vi "STS_show.vi"() -> ()   [LabVIEW 2014]
uses:
  <userlib>/Nanonis Prog Interface V5/Nanonis Prog Interface.lvlib
  <vilib>/Analysis/NI_AALPro.lvlib
panel:
  in  "sub":bool
  in  "Filter order (2) 3":i32=2 min=1 max=1000 step=1
  in  "Filter type (none) 3":T1(ring)
  in  "Display (Y) off":u16(ring) items=["Y", "dY/dX", "dY/dX/(Y/X)"]
  in  "Datafile (1=last) 2":i32
  out "path out 2":path=path "D:/STM Data/092016/160908_16-21-42_STS001.dat"
  in  "Datafile (1=last)":i32
  out "x/y":dbl=-0.00010071572331476725 format="%#_6p"
  in  "fit":dbl=0.0040000000000000036 step=0.001 format="%#_6p"
  out "path out":path=path "D:/STM Data/092016/160908_16-21-42_STS001.dat"
  in  "Filter type pre":T1(ring)=enum."Gaussian"
  in  "Filter order pre":i32=1 min=1 max=1000 step=1
  in  "Ring":u16(ring)=1 items=["Bias calc (V)", "Current (A)", "LI Demod 1 X (A)", "LI Demod 1 Y (A)", "LI Demod 2 X (A)", "LI Demod 2 Y (A)", "Current [bwd] (A)", "LI Demod 1 X [bwd] (A)", "LI Demod 1 Y [bwd] (A)", "LI Demod 2 X [bwd] (A)", "LI Demod 2 Y [bwd] (A)", "Current (A) [filt]", "LI Demod 1 X (A) [filt]", "LI Demod 1 Y (A) [filt]", "LI Demod 2 X (A) [filt]", "LI Demod 2 Y (A) [filt]", "Current (A) [bwd] [filt]", "LI Demod 1 X (A) [bwd] [filt]", "LI Demod 1 Y (A) [bwd] [filt]", "LI Demod 2 X (A) [bwd] [filt]", "LI Demod 2 Y (A) [bwd] [filt]"]
  in  "Filter order (2) 2":i32=2 min=1 max=1000 step=1
  in  "Filter type (none) 2":T1(ring)
  in  "Cutoff frq (0.125) 2":dbl=0.125
  in  "Display (Y) 2":u16(ring)=1 items=["Y", "dY/dX", "dY/dX/(Y/X)"]
  in  "Filter type (none)":T1(ring)
  in  "Filter order (2)":i32=2 min=1 max=1000 step=1
  in  "Cutoff frq (0.125)":dbl=0.125
  in  "Display (Y)":u16(ring)=1 items=["Y", "dY/dX", "dY/dX/(Y/X)"]
  out "XY Graph 3":cluster{"X":dbl, "Y":dbl}[](graph)=[{"X"=-0.029999999329447746, "Y"=nan}, {"X"=-0.02939390018582344, "Y"=nan}, {"X"=-0.028787899762392044, "Y"=1.5525849362798114e-07}, {"X"=-0.02818180061876774, "Y"=5.168520876965395e-07}, {"X"=-0.027575800195336342, "Y"=-1.8705937225910675e-07}, {"X"=-0.026969699189066887, "Y"=-6.639889207903243e-07}, {"X"=-0.02636360004544258, "Y"=-9.874879833106362e-07}, {"X"=-0.025757599622011185, "Y"=-9.458443087316431e-07}, {"X"=-0.02515150047838688, "Y"=6.648643762964484e-07}, {"X"=-0.024545500054955482, "Y"=-4.47928062817252e-08}, {"X"=-0.023939400911331177, "Y"=-1.997370443932008e-06}, {"X"=-0.023333299905061722, "Y"=-2.2367739676225265e-06}, {"X"=-0.022727299481630325, "Y"=5.692607935118802e-07}, {"X"=-0.02212120033800602, "Y"=-1.5689885119641845e-06}, {"X"=-0.021515099331736565, "Y"=-2.758229187147329e-06}, {"X"=-0.020909100770950317, "Y"=-3.194582565724868e-06}, {"X"=-0.020302999764680862, "Y"=-5.236577534894633e-06}, {"X"=-0.019696999341249466, "Y"=-4.579991401925592e-06}, {"X"=-0.01909090019762516, "Y"=-1.7059288454535867e-06}, {"X"=-0.018484799191355705, "Y"=-5.031002994112464e-06}, {"X"=-0.017878800630569458, "Y"=-4.138250071188697e-06}, {"X"=-0.017272699624300003, "Y"=1.3100562902328957e-06}, {"X"=-0.016666699200868607, "Y"=5.068503950570972e-06}, {"X"=-0.0160606000572443, "Y"=4.011176770052973e-06}, {"X"=-0.01545449998229742, "Y"=2.537647009919699e-06}, {"X"=-0.014848499558866024, "Y"=5.116801095124242e-06}, {"X"=-0.014242400415241718, "Y"=1.6464771934735616e-07}, {"X"=-0.013636399991810322, "Y"=-3.0547176995608757e-06}, {"X"=-0.013030299916863441, "Y"=-5.217728993780238e-06}, {"X"=-0.012424199841916561, "Y"=-4.200614920252031e-06}, {"X"=-0.01181820034980774, "Y"=-6.242418446009756e-06}, {"X"=-0.011212100274860859, "Y"=-5.663095474505132e-06}, {"X"=-0.010606099851429462, "Y"=2.384088352720359e-06}, {"X"=-0.009999999776482582, "Y"=5.200079061493491e-06}, {"X"=-0.00939393974840641, "Y"=2.6398627367813077e-06}, {"X"=-0.008787879720330238, "Y"=6.452597551494918e-06}, {"X"=-0.008181819692254066, "Y"=1.2737566183337942e-05}, {"X"=-0.007575760129839182, "Y"=1.218992844152106e-05}, {"X"=-0.00696970010176301, "Y"=1.3279965824539184e-05}, {"X"=-0.006363640073686838, "Y"=1.1414322380559252e-05}, {"X"=-0.005757580045610666, "Y"=9.543383623890207e-06}, {"X"=-0.005151509772986174, "Y"=5.78405585714029e-06}, {"X"=-0.004545450210571289, "Y"=3.834239501672442e-06}, {"X"=-0.003939390182495117, "Y"=3.134550055729865e-06}, {"X"=-0.0033333299215883017, "Y"=1.0710322804966455e-06}, {"X"=-0.00272726989351213, "Y"=-8.661794169541851e-07}, {"X"=-0.0021212100982666016, "Y"=-1.4950962022879021e-06}, {"X"=-0.0015151499537751079, "Y"=-1.4481620816107035e-06}, {"X"=-0.0009090899839065969, "Y"=1.666731229290195e-07}, {"X"=-0.00030303001403808594, "Y"=-1.0913610732735875e-07}, {"X"=0.000303031993098557, "Y"=-1.1114294931287702e-06}, {"X"=0.0009090920211747289, "Y"=-1.284203208185384e-06}, {"X"=0.0015151499537751079, "Y"=6.035322429293407e-07}, {"X"=0.0021212100982666016, "Y"=4.756593350934117e-07}, {"X"=0.00272726989351213, "Y"=2.604464071554455e-07}, {"X"=0.0033333399333059788, "Y"=-1.6241975350996586e-09}, {"X"=0.003939399961382151, "Y"=-6.075334228327941e-07}, {"X"=0.0045454599894583225, "Y"=5.413411018824718e-07}, {"X"=0.005151520017534494, "Y"=-6.982397520424381e-07}, {"X"=0.005757580045610666, "Y"=-2.891121857582741e-06}, {"X"=0.006363640073686838, "Y"=-6.245094796472283e-06}, {"X"=0.00696970010176301, "Y"=-7.859388367794901e-06}, {"X"=0.007575760129839182, "Y"=-9.478467599884328e-06}, {"X"=0.008181819692254066, "Y"=-1.1359428289945348e-05}, {"X"=0.008787879720330238, "Y"=-1.258334103807099e-05}, {"X"=0.00939393974840641, "Y"=-9.133998297466377e-06}, {"X"=0.009999999776482582, "Y"=-8.996086304044726e-06}, {"X"=0.010606099851429462, "Y"=-7.816056623611081e-06}, {"X"=0.011212100274860859, "Y"=-2.158336854899807e-06}, {"X"=0.01181820034980774, "Y"=4.32424257909858e-06}, {"X"=0.012424199841916561, "Y"=2.8658121975906245e-06}, {"X"=0.013030299916863441, "Y"=2.6437646358981405e-06}, {"X"=0.013636399991810322, "Y"=5.652839123077133e-06}, {"X"=0.014242400415241718, "Y"=4.531496689082075e-06}, {"X"=0.014848499558866024, "Y"=3.876928205429419e-06}, {"X"=0.01545449998229742, "Y"=-8.604612293367695e-07}, {"X"=0.0160606000572443, "Y"=-4.179218333770935e-06}, {"X"=0.016666699200868607, "Y"=-4.138505304353997e-06}, {"X"=0.017272699624300003, "Y"=-7.2625928712624055e-06}, {"X"=0.017878800630569458, "Y"=-4.703849285510032e-06}, {"X"=0.018484799191355705, "Y"=-1.8761172247980886e-06}, {"X"=0.01909090019762516, "Y"=2.9486464571849516e-06}, {"X"=0.019696999341249466, "Y"=5.764776470791144e-06}, {"X"=0.020302999764680862, "Y"=3.1401164125217956e-06}, {"X"=0.020909100770950317, "Y"=5.540729187932117e-06}, {"X"=0.021515199914574623, "Y"=5.104789941335857e-06}, {"X"=0.02212120033800602, "Y"=3.022872010196525e-06}, {"X"=0.022727299481630325, "Y"=1.5019503969055098e-06}, {"X"=0.023333299905061722, "Y"=2.6840593826798465e-06}, {"X"=0.023939400911331177, "Y"=3.009385765408917e-06}, {"X"=0.024545500054955482, "Y"=6.751681966771312e-07}, {"X"=0.02515150047838688, "Y"=2.3592434760700652e-07}, {"X"=0.025757599622011185, "Y"=1.0180363796469083e-06}, {"X"=0.02636360004544258, "Y"=7.318487219108044e-07}, {"X"=0.026969699189066887, "Y"=7.621898569330085e-07}, {"X"=0.027575800195336342, "Y"=5.613791177103256e-07}, {"X"=0.02818180061876774, "Y"=-3.547310154327501e-07}, {"X"=0.028787899762392044, "Y"=4.214083566107483e-07}, {"X"=0.02939390018582344, "Y"=7.204319939562927e-07}, {"X"=0.029999999329447746, "Y"=8.404090983124726e-07}]
  out "XY Graph 2":cluster{"X":dbl, "Y":dbl}[](graph)=[{"X"=-0.029999999329447746, "Y"=nan}, {"X"=-0.02939390018582344, "Y"=3.391442095720389e-08}, {"X"=-0.028787899762392044, "Y"=3.400850767008377e-08}, {"X"=-0.02818180061876774, "Y"=3.432177127781708e-08}, {"X"=-0.027575800195336342, "Y"=3.420841321902125e-08}, {"X"=-0.026969699189066887, "Y"=3.380596886597846e-08}, {"X"=-0.02636360004544258, "Y"=3.320745324495459e-08}, {"X"=-0.025757599622011185, "Y"=3.263427119336304e-08}, {"X"=-0.02515150047838688, "Y"=3.3037244922462626e-08}, {"X"=-0.024545500054955482, "Y"=3.301010046288922e-08}, {"X"=-0.023939400911331177, "Y"=3.179949594732153e-08}, {"X"=-0.023333299905061722, "Y"=3.0443784994748196e-08}, {"X"=-0.022727299481630325, "Y"=3.078875727665929e-08}, {"X"=-0.02212120033800602, "Y"=2.983779468320142e-08}, {"X"=-0.021515099331736565, "Y"=2.8166029197349645e-08}, {"X"=-0.020909100770950317, "Y"=2.623011676020754e-08}, {"X"=-0.020302999764680862, "Y"=2.305622184689988e-08}, {"X"=-0.019696999341249466, "Y"=2.0280745118020816e-08}, {"X"=-0.01909090019762516, "Y"=1.9246783105707396e-08}, {"X"=-0.018484799191355705, "Y"=1.619748712843119e-08}, {"X"=-0.017878800630569458, "Y"=1.3689713541117256e-08}, {"X"=-0.017272699624300003, "Y"=1.4483739976897043e-08}, {"X"=-0.016666699200868607, "Y"=1.7555255517106758e-08}, {"X"=-0.0160606000572443, "Y"=1.9986426322361574e-08}, {"X"=-0.01545449998229742, "Y"=2.152449436526263e-08}, {"X"=-0.014848499558866024, "Y"=2.4625277995522153e-08}, {"X"=-0.014242400415241718, "Y"=2.472507083721828e-08}, {"X"=-0.013636399991810322, "Y"=2.287391061782101e-08}, {"X"=-0.013030299916863441, "Y"=1.9711444683638296e-08}, {"X"=-0.012424199841916561, "Y"=1.7165451665650556e-08}, {"X"=-0.01181820034980774, "Y"=1.3382549257837903e-08}, {"X"=-0.011212100274860859, "Y"=9.950146666309003e-09}, {"X"=-0.010606099851429462, "Y"=1.1394905217555401e-08}, {"X"=-0.009999999776482582, "Y"=1.454667352645631e-08}, {"X"=-0.00939393974840641, "Y"=1.614658881082723e-08}, {"X"=-0.008787879720330238, "Y"=2.0057250264050477e-08}, {"X"=-0.008181819692254066, "Y"=2.7776979982746367e-08}, {"X"=-0.007575760129839182, "Y"=3.516480267988338e-08}, {"X"=-0.00696970010176301, "Y"=4.32132591403542e-08}, {"X"=-0.006363640073686838, "Y"=5.0131023682786414e-08}, {"X"=-0.005757580045610666, "Y"=5.591488702982299e-08}, {"X"=-0.005151509772986174, "Y"=5.94204313400353e-08}, {"X"=-0.004545450210571289, "Y"=6.174420885461277e-08}, {"X"=-0.003939390182495117, "Y"=6.364393434939458e-08}, {"X"=-0.0033333299215883017, "Y"=6.4293044452752e-08}, {"X"=-0.00272726989351213, "Y"=6.376808773099374e-08}, {"X"=-0.0021212100982666016, "Y"=6.286197003276277e-08}, {"X"=-0.0015151499537751079, "Y"=6.198429671233468e-08}, {"X"=-0.0009090899839065969, "Y"=6.208531062019493e-08}, {"X"=-0.00030303001403808594, "Y"=6.201916759427655e-08}, {"X"=0.000303031993098557, "Y"=6.134557240488006e-08}, {"X"=0.0009090920211747289, "Y"=6.056726817247172e-08}, {"X"=0.0015151499537751079, "Y"=6.093304367587914e-08}, {"X"=0.0021212100982666016, "Y"=6.122132184123459e-08}, {"X"=0.00272726989351213, "Y"=6.137916793742765e-08}, {"X"=0.0033333399333059788, "Y"=6.137818355996292e-08}, {"X"=0.003939399961382151, "Y"=6.100998183666366e-08}, {"X"=0.0045454599894583225, "Y"=6.133806704006934e-08}, {"X"=0.005151520017534494, "Y"=6.09148918363426e-08}, {"X"=0.005757580045610666, "Y"=5.916269844216437e-08}, {"X"=0.006363640073686838, "Y"=5.537779611447602e-08}, {"X"=0.00696970010176301, "Y"=5.0614534979628706e-08}, {"X"=0.007575760129839182, "Y"=4.4870014639923725e-08}, {"X"=0.008181819692254066, "Y"=3.798552450123619e-08}, {"X"=0.008787879720330238, "Y"=3.035926447841084e-08}, {"X"=0.00939393974840641, "Y"=2.482351321380066e-08}, {"X"=0.009999999776482582, "Y"=1.9371344895795647e-08}, {"X"=0.010606099851429462, "Y"=1.463403239043591e-08}, {"X"=0.011212100274860859, "Y"=1.3326079342459039e-08}, {"X"=0.01181820034980774, "Y"=1.594700309373918e-08}, {"X"=0.012424199841916561, "Y"=1.7683683829958364e-08}, {"X"=0.013030299916863441, "Y"=1.928606977391814e-08}, {"X"=0.013636399991810322, "Y"=2.2712255990077847e-08}, {"X"=0.014242400415241718, "Y"=2.5458344902439555e-08}, {"X"=0.014848499558866024, "Y"=2.7808147767643243e-08}, {"X"=0.01545449998229742, "Y"=2.728670789831886e-08}, {"X"=0.0160606000572443, "Y"=2.475368335300092e-08}, {"X"=0.016666699200868607, "Y"=2.2245338832147316e-08}, {"X"=0.017272699624300003, "Y"=1.7844204476952457e-08}, {"X"=0.017878800630569458, "Y"=1.499319669166497e-08}, {"X"=0.018484799191355705, "Y"=1.385627235357104e-08}, {"X"=0.01909090019762516, "Y"=1.5643449938403702e-08}, {"X"=0.019696999341249466, "Y"=1.9137476020535762e-08}, {"X"=0.020302999764680862, "Y"=2.1040387896147848e-08}, {"X"=0.020909100770950317, "Y"=2.4398629432420044e-08}, {"X"=0.021515199914574623, "Y"=2.7492638244245676e-08}, {"X"=0.02212120033800602, "Y"=2.9324499962403687e-08}, {"X"=0.022727299481630325, "Y"=3.02348308117343e-08}, {"X"=0.023333299905061722, "Y"=3.18613719341533e-08}, {"X"=0.023939400911331177, "Y"=3.368536367482062e-08}, {"X"=0.024545500054955482, "Y"=3.4094582540629e-08}, {"X"=0.02515150047838688, "Y"=3.423755279517662e-08}, {"X"=0.025757599622011185, "Y"=3.4854583773059e-08}, {"X"=0.02636360004544258, "Y"=3.529808440842467e-08}, {"X"=0.026969699189066887, "Y"=3.57600470279909e-08}, {"X"=0.027575800195336342, "Y"=3.610029947613379e-08}, {"X"=0.02818180061876774, "Y"=3.588533233057729e-08}, {"X"=0.028787899762392044, "Y"=3.614074757463519e-08}, {"X"=0.02939390018582344, "Y"=3.657732966802623e-08}, {"X"=0.029999999329447746, "Y"=3.7086700902807496e-08}]
  out "XY Graph":cluster{"X":dbl, "Y":dbl}[](graph)=[{"X"=-0.029999999329447746, "Y"=-1.0017100482428987e-09}, {"X"=-0.02939390018582344, "Y"=-9.811545467442232e-10}, {"X"=-0.028787899762392044, "Y"=-9.605453766958825e-10}, {"X"=-0.02818180061876774, "Y"=-9.397429805167283e-10}, {"X"=-0.027575800195336342, "Y"=-9.190126676210852e-10}, {"X"=-0.026969699189066887, "Y"=-8.985228358735018e-10}, {"X"=-0.02636360004544258, "Y"=-8.783958268997907e-10}, {"X"=-0.025757599622011185, "Y"=-8.586194447382376e-10}, {"X"=-0.02515150047838688, "Y"=-8.385955988830266e-10}, {"X"=-0.024545500054955482, "Y"=-8.185914640250028e-10}, {"X"=-0.023939400911331177, "Y"=-7.993178167636466e-10}, {"X"=-0.023333299905061722, "Y"=-7.808658080436788e-10}, {"X"=-0.022727299481630325, "Y"=-7.622078080970968e-10}, {"X"=-0.02212120033800602, "Y"=-7.441231462919706e-10}, {"X"=-0.021515099331736565, "Y"=-7.270516876528421e-10}, {"X"=-0.020909100770950317, "Y"=-7.111562746469011e-10}, {"X"=-0.020302999764680862, "Y"=-6.971818753847233e-10}, {"X"=-0.019696999341249466, "Y"=-6.848917352556985e-10}, {"X"=-0.01909090019762516, "Y"=-6.732262764978065e-10}, {"X"=-0.018484799191355705, "Y"=-6.634089632502278e-10}, {"X"=-0.017878800630569458, "Y"=-6.551130165467347e-10}, {"X"=-0.017272699624300003, "Y"=-6.463344071721923e-10}, {"X"=-0.016666699200868607, "Y"=-6.356959148953792e-10}, {"X"=-0.0160606000572443, "Y"=-6.235821590172856e-10}, {"X"=-0.01545449998229742, "Y"=-6.105361613693062e-10}, {"X"=-0.014848499558866024, "Y"=-5.956132324769039e-10}, {"X"=-0.014242400415241718, "Y"=-5.806273882164156e-10}, {"X"=-0.013636399991810322, "Y"=-5.667657886964842e-10}, {"X"=-0.013030299916863441, "Y"=-5.548186805964197e-10}, {"X"=-0.012424199841916561, "Y"=-5.444146990553719e-10}, {"X"=-0.01181820034980774, "Y"=-5.363048810020008e-10}, {"X"=-0.011212100274860859, "Y"=-5.302740963618185e-10}, {"X"=-0.010606099851429462, "Y"=-5.233687789750193e-10}, {"X"=-0.009999999776482582, "Y"=-5.145520390604063e-10}, {"X"=-0.00939393974840641, "Y"=-5.04766236992382e-10}, {"X"=-0.008787879720330238, "Y"=-4.926103393342207e-10}, {"X"=-0.008181819692254066, "Y"=-4.757758220660062e-10}, {"X"=-0.007575760129839182, "Y"=-4.544638571414303e-10}, {"X"=-0.00696970010176301, "Y"=-4.2827402809356435e-10}, {"X"=-0.006363640073686838, "Y"=-3.978916184728876e-10}, {"X"=-0.005757580045610666, "Y"=-3.6400384046971707e-10}, {"X"=-0.005151509772986174, "Y"=-3.2799088344799693e-10}, {"X"=-0.004545450210571289, "Y"=-2.905702152479171e-10}, {"X"=-0.003939390182495117, "Y"=-2.5199817060924496e-10}, {"X"=-0.0033333299215883017, "Y"=-2.130327113137166e-10}, {"X"=-0.00272726989351213, "Y"=-1.7438542227310674e-10}, {"X"=-0.0021212100982666016, "Y"=-1.3628730958632e-10}, {"X"=-0.0015151499537751079, "Y"=-9.872109776463883e-11}, {"X"=-0.0009090899839065969, "Y"=-6.109367628088635e-11}, {"X"=-0.00030303001403808594, "Y"=-2.3506341437428975e-11}, {"X"=0.000303031993098557, "Y"=1.367287930321889e-11}, {"X"=0.0009090920211747289, "Y"=5.038027955232413e-11}, {"X"=0.0015151499537751079, "Y"=8.730923402957604e-11}, {"X"=0.0021212100982666016, "Y"=1.2441303719063492e-10}, {"X"=0.00272726989351213, "Y"=1.616124831431332e-10}, {"X"=0.0033333399333059788, "Y"=1.988119612957941e-10}, {"X"=0.003939399961382151, "Y"=2.357876726006492e-10}, {"X"=0.0045454599894583225, "Y"=2.7296222323309175e-10}, {"X"=0.005151520017534494, "Y"=3.098803042896825e-10}, {"X"=0.005757580045610666, "Y"=3.4573645096860274e-10}, {"X"=0.006363640073686838, "Y"=3.792987196365386e-10}, {"X"=0.00696970010176301, "Y"=4.0997416612735476e-10}, {"X"=0.007575760129839182, "Y"=4.371680884598052e-10}, {"X"=0.008181819692254066, "Y"=4.6018957881712426e-10}, {"X"=0.008787879720330238, "Y"=4.785891154992819e-10}, {"X"=0.00939393974840641, "Y"=4.936336546145871e-10}, {"X"=0.009999999776482582, "Y"=5.053738524460062e-10}, {"X"=0.010606099851429462, "Y"=5.142435405746245e-10}, {"X"=0.011212100274860859, "Y"=5.223191502988351e-10}, {"X"=0.01181820034980774, "Y"=5.319846300691285e-10}, {"X"=0.012424199841916561, "Y"=5.427009334886963e-10}, {"X"=0.013030299916863441, "Y"=5.543902218240988e-10}, {"X"=0.013636399991810322, "Y"=5.681561218818977e-10}, {"X"=0.014242400415241718, "Y"=5.835838896726386e-10}, {"X"=0.014848499558866024, "Y"=6.004383842203854e-10}, {"X"=0.01545449998229742, "Y"=6.169741407608154e-10}, {"X"=0.0160606000572443, "Y"=6.319773500962806e-10}, {"X"=0.016666699200868607, "Y"=6.454602309120776e-10}, {"X"=0.017272699624300003, "Y"=6.562738263809072e-10}, {"X"=0.017878800630569458, "Y"=6.653612179829212e-10}, {"X"=0.018484799191355705, "Y"=6.737580990870476e-10}, {"X"=0.01909090019762516, "Y"=6.832396098362399e-10}, {"X"=0.019696999341249466, "Y"=6.948388176634173e-10}, {"X"=0.020302999764680862, "Y"=7.075893016376437e-10}, {"X"=0.020909100770950317, "Y"=7.22377335488229e-10}, {"X"=0.021515199914574623, "Y"=7.390405999840392e-10}, {"X"=0.02212120033800602, "Y"=7.568112593781698e-10}, {"X"=0.022727299481630325, "Y"=7.751365644407877e-10}, {"X"=0.023333299905061722, "Y"=7.944445693239898e-10}, {"X"=0.023939400911331177, "Y"=8.148613021438512e-10}, {"X"=0.024545500054955482, "Y"=8.355259994239546e-10}, {"X"=0.02515150047838688, "Y"=8.562739709150864e-10}, {"X"=0.025757599622011185, "Y"=8.773993042913191e-10}, {"X"=0.02636360004544258, "Y"=8.987899583891416e-10}, {"X"=0.026969699189066887, "Y"=9.204640922687718e-10}, {"X"=0.027575800195336342, "Y"=9.423445201078852e-10}, {"X"=0.02818180061876774, "Y"=9.640910466951914e-10}, {"X"=0.028787899762392044, "Y"=9.8599592285012e-10}, {"X"=0.02939390018582344, "Y"=1.0081618001169337e-09}, {"X"=0.029999999329447746, "Y"=1.030640017773976e-09}]
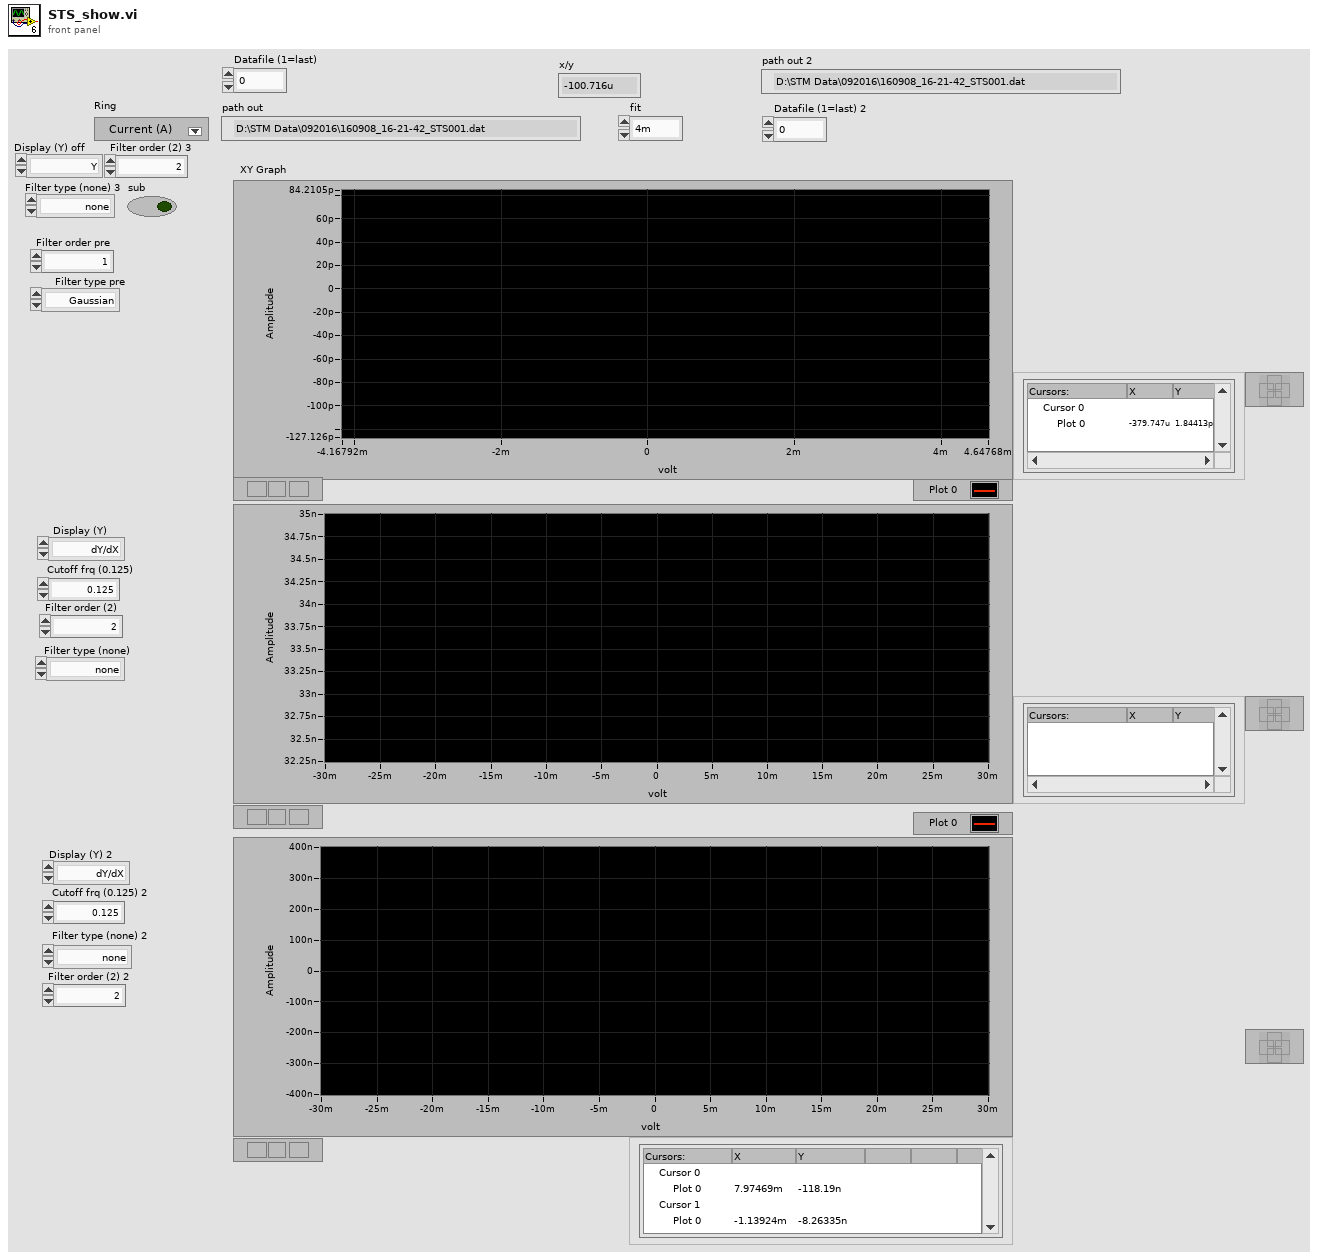
[diagram p1: front panel]
types:
  T1 = enum16{"none", "Gaussian", "Butterworth", "5th order FIR"}
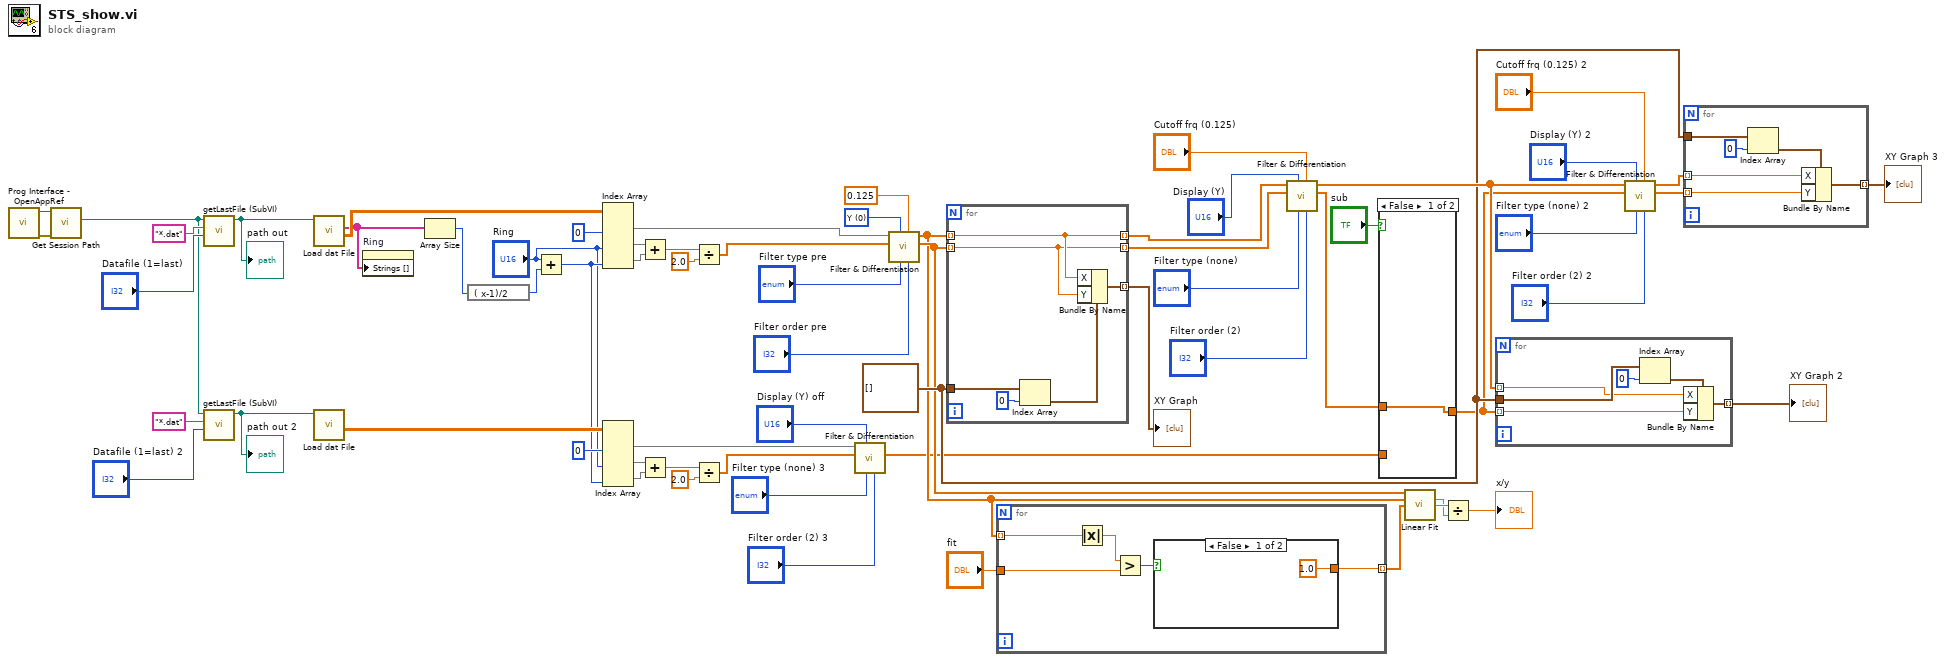
[diagram p0: block diagram]
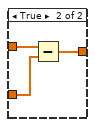
[diagram p2: hidden frame]
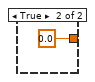
[diagram p3: hidden frame]
diagram:
  w35 = u16 0 items=["Y", "dY/dX", "dY/dX/(Y/X)"] ("Display (Y)")
  w44 = cluster{"X":dbl, "Y":dbl}[] [] ("XY Graph")
  n1 = call <userlib>:"Prog Interface - OpenAppRef.vi"() -> ("Error out"=w60:errorcluster, "Application reference"=w59:refnum<vi>)  [unwired: 6 in]
  n2 = call <userlib>:"Get Session Path.vi"("error in (no error)"=w60, "Application ref in"=w59) -> ("Session path"=w54:path)  [unwired: 7 in, 2 out]
  n3 = call "getLastFile (SubVI).vi"("Datafile (1=last)"="Datafile (1=last)", "pattern"="*.dat", "Session path"=w54) -> ("path out"=w58:path)  [unwired: 8 in]
  "path out" <- w58
  n4 = call "getLastFile (SubVI).vi"("Datafile (1=last)"="Datafile (1=last) 2", "pattern"="*.dat", "Session path"=w54) -> ("path out"=w53:path)  [unwired: 8 in]
  "path out 2" <- w53
  n5 = call <userlib>:"Load dat File.vi"("File path"=w58) -> ("Data"=w65:sgl[][], "Channels names"=w64:string[])  [unwired: 7 in, 2 out]
  n6 = call <userlib>:"Load dat File.vi"("File path"=w53) -> ("Data"=w52:sgl[][])  [unwired: 7 in, 3 out]
  n7 = property on="Ring" class="Ring (strict)"("Strings []"=w64) -> ()  [unwired: 2 in, 2 out]
  n8 = Array Size(array=w64) -> (size(s)=w63:i32)
  n9 = expression code="( x-1)/2"(w63) -> (w62:i32)
  n10 = Add(x="Ring", y=w62) -> (x+y=w16:i32)
  n11 = Index Array(array=w65, index (col) #1=0 ("index (row)"), index (col) #2="Ring", index (col) #3=w16) -> (element #1=w29:sgl[], element #2=w31:sgl[], element #3=w30:sgl[])  [unwired: 3 in]
  n12 = Index Array(array=w52, index (col) #1=0 ("index (row)"), index (col) #2="Ring", index (col) #3=w16) -> (element #1=w9:sgl[], element #2=w12:sgl[], element #3=w11:sgl[])  [unwired: 3 in]
  n13 = Add(x=w31, y=w30) -> (x+y=w26:sgl[])
  n14 = Add(x=w12, y=w11) -> (x+y=w14:sgl[])
  n15 = Divide(x=w26, y=2.0 ("Cutoff frq (0.125)")) -> (x/y=w27:dbl[])
  n16 = Divide(x=w14, y=2.0 ("Cutoff frq (0.125)")) -> (x/y=w10:dbl[])
  n17 = call <userlib>:"Filter & Differentiation.vi"("Filter order (2)"="Filter order (2) 3", "Filter type (none)"="Filter type (none) 3", "Display (Y)"="Display (Y) off", "Y in"=w10, "X in"=w9) -> ("Y out"=w1:dbl[])  [unwired: 4 in, 2 out]
  n18 = call <userlib>:"Filter & Differentiation.vi"("Filter order (2)"="Filter order pre", "Cutoff frq (0.125)"=0.125, "Filter type (none)"="Filter type pre", "Display (Y)"=w35, "Y in"=w27, "X in"=w29) -> ("Y out"=w24:dbl[], "X out"=w22:dbl[])  [unwired: 3 in, 1 out]
  n19 = for {
    tunnel: w44 -> [w71]
    tunnel: w22 -> [w67] mode=indexing
    tunnel: w24 -> [w66] mode=indexing
    tunnel: [w68] -> w51 mode=indexing
    tunnel: [w67] -> w50 mode=indexing
    tunnel: [w66] -> w49 mode=indexing
    n20 = Index Array(array=w71, index=0) -> (element=w70:cluster{"X":dbl, "Y":dbl})
    n21 = Bundle By Name(cluster=w70, "X"=w67, "Y"=w66) -> (w68:cluster{"X":dbl, "Y":dbl})
  }
  "XY Graph" <- w51
  n22 = for {
    tunnel: "fit" -> [w76]
    tunnel: w22 -> [w74] mode=indexing
    tunnel: [w73] -> w21 mode=indexing
    n23 = Absolute Value(x=w74) -> (abs(x)=w72:dbl)
    n24 = Greater?(x=w72, y=w76) -> (0:w75:bool)
    n25 = case shown="False" w75 {
      tunnel: [1.0 0.0] -> w73
      frame False {
      }
      frame True {
      }
    }
  }
  n26 = call <userlib>:"Filter & Differentiation.vi"("Filter order (2)"="Filter order (2)", "Cutoff frq (0.125)"="Cutoff frq (0.125)", "Filter type (none)"="Filter type (none)", "Display (Y)"="Display (Y)", "Y in"=w49, "X in"=w50) -> ("Y out"=w4:dbl[], "X out"=w47:dbl[])  [unwired: 3 in, 1 out]
  n27 = case shown="False" "sub" {
    tunnel: w1 -> [_ w80]
    tunnel: [w79 w81] -> w3
    tunnel: w4 -> [w79 w82]
    frame False {
    }
    frame True {
      n28 = Subtract(x=w82, y=w80) -> (x-y=w81:dbl[])
    }
  }
  n29 = call <vilib>:"Linear Fit.vi"("Y"=w24, "X"=w22, "Weight"=w21) -> ("slope"=w19:dbl, "intercept"=w20:dbl)  [unwired: 8 in, 3 out]
  n30 = Divide(x=w20, y=w19) -> (x/y=→"x/y":dbl)
  n31 = for {
    tunnel: w44 -> [w88]
    tunnel: w47 -> [w84] mode=indexing
    tunnel: w3 -> [w83] mode=indexing
    tunnel: [w85] -> w2 mode=indexing
    n32 = Index Array(array=w88, index=0) -> (element=w87:cluster{"X":dbl, "Y":dbl})
    n33 = Bundle By Name(cluster=w87, "X"=w84, "Y"=w83) -> (w85:cluster{"X":dbl, "Y":dbl})
  }
  "XY Graph 2" <- w2
  n34 = call <userlib>:"Filter & Differentiation.vi"("Filter order (2)"="Filter order (2) 2", "Cutoff frq (0.125)"="Cutoff frq (0.125) 2", "Filter type (none)"="Filter type (none) 2", "Display (Y)"="Display (Y) 2", "Y in"=w3, "X in"=w47) -> ("Y out"=w45:dbl[], "X out"=w46:dbl[])  [unwired: 3 in, 1 out]
  n35 = for {
    tunnel: w44 -> [w94]
    tunnel: w46 -> [w90] mode=indexing
    tunnel: w45 -> [w89] mode=indexing
    tunnel: [w91] -> w48 mode=indexing
    n36 = Index Array(array=w94, index=0) -> (element=w93:cluster{"X":dbl, "Y":dbl})
    n37 = Bundle By Name(cluster=w93, "X"=w90, "Y"=w89) -> (w91:cluster{"X":dbl, "Y":dbl})
  }
  "XY Graph 3" <- w48
